vi "SetAnalogOutput.vi"(2 "Reference Clock Properties":T1={"RefClockGlobalName"="/PXI1Slot2/PXI_Clk10", "RefClockRate"=100000.0}, 3 "Error In":errorcluster, 4 "Analog Output Voltage Setup":T2=[{"AnalogOut (Volt)"=[5.0, 5.0, 5.0, 5.0], "DAQmx Device Name"="PXI1Slot2"}, {"AnalogOut (Volt)"=[5.0, 5.0, 5.0, 5.0], "DAQmx Device Name"="PXI1Slot3"}, {"AnalogOut (Volt)"=[5.0, 5.0, 5.0, 5.0], "DAQmx Device Name"="PXI1Slot6"}]) -> (0 "Error Out":errorcluster, 1 "AnalogTaskOut":refnum<k21>[](array[refnum]))   [LabVIEW 2012]
uses:
  controls/AnalogOutputSetup.ctl
  controls/RefClockSettings.ctl
  <vilib>/DAQmx/write.llb/DAQmx Write (Analog 1D DBL NChan 1Samp).vi
  <vilib>/DAQmx/create/channels.llb/DAQmx Create Channel (AO-Voltage-Basic).vi
  <vilib>/DAQmx/miscellaneous.llb/DAQmx Fill In Error Info.vi
  <resource>/objmgr/daqmx.rc
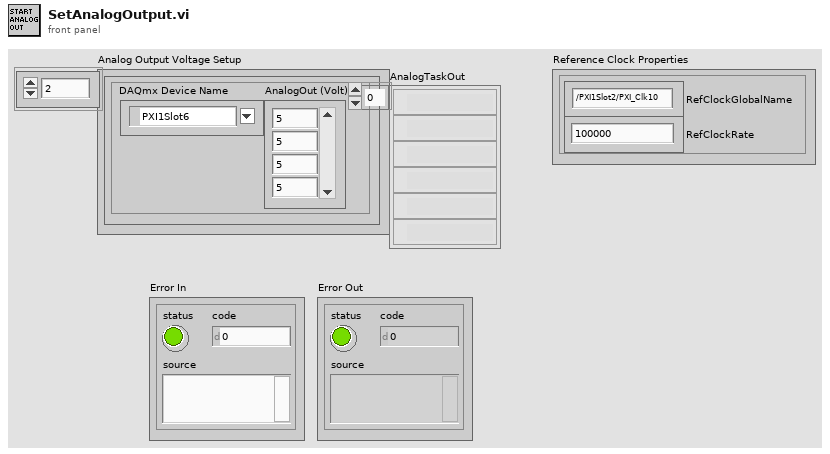
[diagram p1: front panel]
types:
  T1 = typedef "RefClockSettings.ctl" = cluster{"RefClockGlobalName":string, "RefClockRate":dbl}
  T2 = typedef "AnalogOutputSetup.ctl" = cluster{"AnalogOut (Volt)":dbl[], "DAQmx Device Name":tag}[]
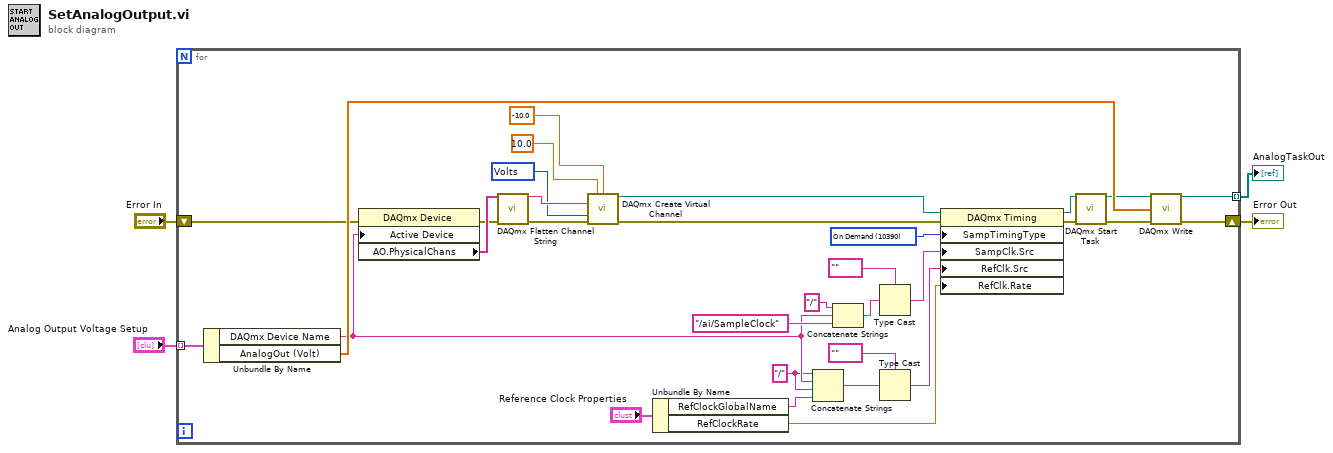
[diagram p0: block diagram]
diagram:
  n1 = for {
    tunnel: "Analog Output Voltage Setup" -> [w36] mode=indexing
    shift-right: [w18] -> w2
    shift-left: "Error In" -> [w29]
    tunnel: [w19] -> w1 mode=indexing
    w7 = "/"
    w17 = 10390 items=["Sample Clock"=10388, "Burst Handshake"=12548, "Handshake"=10389, "Implicit"=10451, "On Demand"=10390, "Change Detection"=12504, "Pipelined Sample Clock"=14668] ("SampTimingType")
    w32 = 10348 items=["Volts"=10348, "From Custom Scale"=10065] ("units")
    n2 = Unbundle By Name(w36) -> ("DAQmx Device Name"=w9:tag, "AnalogOut (Volt)"=w31:dbl[])
    n3 = property class="DAQmx Device"(error in=w29, "Active Device"=w9) -> (error out=w28:errorcluster, "AO.PhysicalChans"=w30:tag[])  [unwired: 1 in, 1 out]
    n4 = call <vilib>:"DAQmx Flatten Channel String.vi"("names in"=w30, "error in"=w28) -> ("names out"=w35:string, "error out"=w27:errorcluster)  [unwired: 12 in]
    n5 = call-poly <vilib>:"DAQmx Create Virtual Channel.vi"("maximum value"=10.0, "minimum value"=-10.0 ("maximum value"), "physical channels"=w35, "units"=w32, "error in"=w27) -> ("task out"=w16:refnum<k21>, "error out"=w14:errorcluster)  [unwired: 9 in]
    n6 = Unbundle By Name("Reference Clock Properties") -> ("RefClockGlobalName"=w6:string, "RefClockRate"=w5:dbl)
    n7 = Concatenate Strings(w7, w9, w7, w6) -> (w10:string)
    n8 = Concatenate Strings("/", w9, "/ai/SampleClock" ("string")) -> (w23:string)
    n9 = Type Cast(type=tag "", x=w23) -> (*(type *) &x=w12:tag)
    n10 = Type Cast(type=tag "", x=w10) -> (*(type *) &x=w8:tag)
    n11 = property class="DAQmx Timing"(reference=w16, error in=w14, "SampTimingType"=w17, "SampClk.Src"=w12, "RefClk.Src"=w8, "RefClk.Rate"=w5) -> (reference out=w15:refnum<k21>, error out=w13:errorcluster)
    n12 = call <vilib>:"DAQmx Start Task.vi"("task/channels in"=w15, "error in"=w13) -> ("task out"=w20:refnum<k21>, "error out"=w21:errorcluster)  [unwired: 12 in]
    n13 = call-poly <vilib>:"DAQmx Write.vi"("task/channels in"=w20, "data"=w31, "error in"=w21) -> ("task out"=w19:refnum<k21>, "error out"=w18:errorcluster)  [unwired: 10 in, 1 out]
  }
  "Error Out" <- w2
  "AnalogTaskOut" <- w1
